vi "WPI_RelaySet.vi"(8 "error in (no error)":errorcluster, 10 "RelayValue":T1, 11 "RelayDevRef":T2={"DevStatus"={"status"=FALSE, "code"=0, "source"=""}, "Relay Channel"=enum."Invalid", "Relay Direction"=enum."Both directions"}) -> (0 "error out":errorcluster, 3 "RelayDevRef":T2={"DevStatus"={"status"=FALSE, "code"=0, "source"=""}, "Relay Channel"=enum."Invalid", "Relay Direction"=enum."Both directions"})   [LabVIEW 2017]
doc: "Specifies the direction of the motors corresponding to the relay you specify.\n\nThis software is licensed. Open the labview\\readme\\WPI Robotics Library Open Source License.txt file for more information."
uses:
  <vilib>/Rock Robotics/WPI/Relay/WPI_RelayDevRef.ctl
  <vilib>/Rock Robotics/SystemInterfaces/DIO/FPGA_DIORelayChannel.ctl
  <vilib>/Rock Robotics/WPI/Relay/WPI_RelayDirection.ctl
  <vilib>/Rock Robotics/WPI/Relay/WPI_RelayValue.ctl
  <vilib>/Rock Robotics/WPI/Relay/WPI_RelayCacheOp.ctl
  <vilib>/Rock Robotics/WPI/Relay/WPI_RelaySafetyCheck.vi
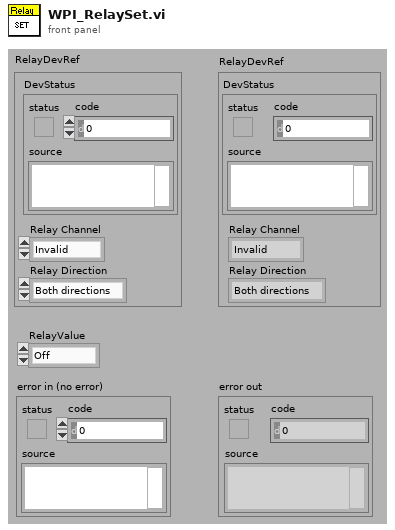
[diagram p1: front panel]
types:
  T1 = typedef "WPI_RelayValue.ctl" = enum16{"Off", "On", "Forward", "Reverse"}
  T2 = typedef "WPI_RelayDevRef.ctl" = cluster{"DevStatus":errorcluster, "Relay Channel":T3, "Relay Direction":T4}
  T3 = typedef "FPGA_DIORelayChannel.ctl" = enum8{"Relay 0", "Relay 1", "Relay 2", "Relay 3", "Invalid"}
  T4 = typedef "WPI_RelayDirection.ctl" = enum16{"Both directions", "Forward only", "Reverse only"}
  T5 = typedef "WPI_RelayCacheOp.ctl" = enum16{"Acquire", "Release", "Status"}
  T6 = typedef "WPI_DigitalModuleDeviceRef.ctl" = cluster{"DevStatus":errorcluster}
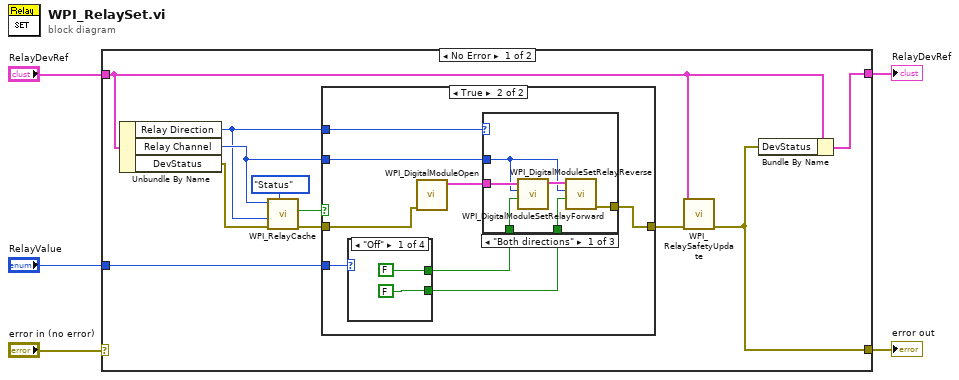
[diagram p0: block diagram]
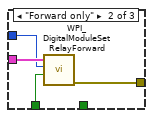
[diagram p3: hidden frame]
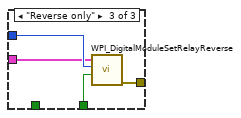
[diagram p4: hidden frame]
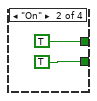
[diagram p5: hidden frame]
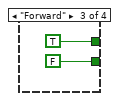
[diagram p6: hidden frame]
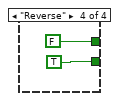
[diagram p7: hidden frame]
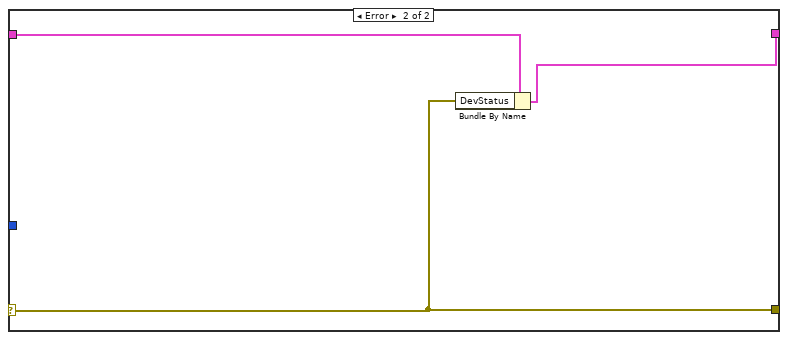
[diagram p8: hidden frame]
diagram:
  n1 = case shown="No Error" "error in (no error)" {
    selector: "error in (no error)" -> [_ w48]
    tunnel: "RelayValue" -> [w16 _]
    tunnel: "RelayDevRef" -> [w6 w49]
    tunnel: [w15 w50] -> w2
    tunnel: [w7 w48] -> w1
    frame No Error {
      n2 = Unbundle By Name(w6) -> ("Relay Direction"=w9:T4, "Relay Channel"=w13:T3, "DevStatus"=w12:errorcluster)
      n3 = call <vilib>:"WPI_RelayCache.vi"("Operation"=WPI_RelayCacheOp."Status", "error in (no error)"=w12, "RelayDirection"=w9, "RelayChannelIn"=w13) -> ("error out"=w10:errorcluster, "Allocated"=w11:bool)  [unwired: 1 in, 5 out]
      n4 = case shown="True" w11 {
        tunnel: w16 -> [_ w25]
        tunnel: [w17 w20] -> w8
        tunnel: w13 -> [_ w18]
        tunnel: w10 -> [w17 w23]
        tunnel: w9 -> [_ w19]
        frame False {
        }
        frame True {
          n5 = case shown="\"Off\"" w25 {
            tunnel: [FALSE TRUE TRUE FALSE] -> w22
            tunnel: [FALSE TRUE FALSE TRUE] -> w21
            frame "Off" {
            }
            frame "On" {
            }
            frame "Forward" {
            }
            frame "Reverse" {
            }
          }
          n6 = call <vilib>:"WPI_DigitalModuleOpen.vi"("error in (no error)"=w23) -> ("DigitalModuleDevRef"=w24:T6)  [unwired: 1 in, 9 out]
          n7 = case shown="\"Both directions\"" w19 {
            tunnel: w24 -> [w30 w35 w36]
            tunnel: w22 -> [w29 w34 _]
            tunnel: w21 -> [w28 _ w39]
            tunnel: [w27 w32 w38] -> w20
            tunnel: w18 -> [w26 w33 w37]
            frame "Both directions" {
              n8 = call <vilib>:"WPI_DigitalModuleSetRelayForward.vi"("Value"=w29, "RelayChannel"=w26, "DigitalModuleDevRef"=w30) -> ("DigitalModuleDevRef"=w31:T6)  [unwired: 1 in, 7 out]
              n9 = call <vilib>:"WPI_DigitalModuleSetRelayReverse.vi"("Value"=w28, "RelayChannel"=w26, "DigitalModuleDevRef"=w31) -> ("error out"=w27:errorcluster)  [unwired: 1 in, 7 out]
            }
            frame "Forward only" {
              n10 = call <vilib>:"WPI_DigitalModuleSetRelayForward.vi"("Value"=w34, "RelayChannel"=w33, "DigitalModuleDevRef"=w35) -> ("error out"=w32:errorcluster)  [unwired: 1 in, 7 out]
            }
            frame "Reverse only" {
              n11 = call <vilib>:"WPI_DigitalModuleSetRelayReverse.vi"("Value"=w39, "RelayChannel"=w37, "DigitalModuleDevRef"=w36) -> ("error out"=w38:errorcluster)  [unwired: 1 in, 7 out]
            }
          }
        }
      }
      n12 = call <vilib>:"WPI_RelaySafetyUpdate.vi"("error in (no error)"=w8, "RelayDevRef"=w6) -> ("error out"=w7:errorcluster)  [unwired: 9 out]
      n13 = Bundle By Name(cluster=w6, "DevStatus"=w7) -> (w15:T2)
    }
    frame Error {
      n14 = Bundle By Name(cluster=w49, "DevStatus"=w48) -> (w50:T2)
    }
  }
  "RelayDevRef" <- w2
  "error out" <- w1
